vi "IG Create Error.vi"(4 "Skip Call Stack (1)":i32=1, 5 "Is Warning? (F)":bool, 6 "Name (Immediate Caller)":string, 7 "Show Call Chain? (T)":bool=TRUE, 8 "error in (no error)":errorcluster, 10 "Message (\"\")":string, 11 "Code":i32=1) -> (0 "error out":errorcluster)   [LabVIEW 2020, in "WS Admin.lvlib"]
uses:
  WS Admin.lvlib
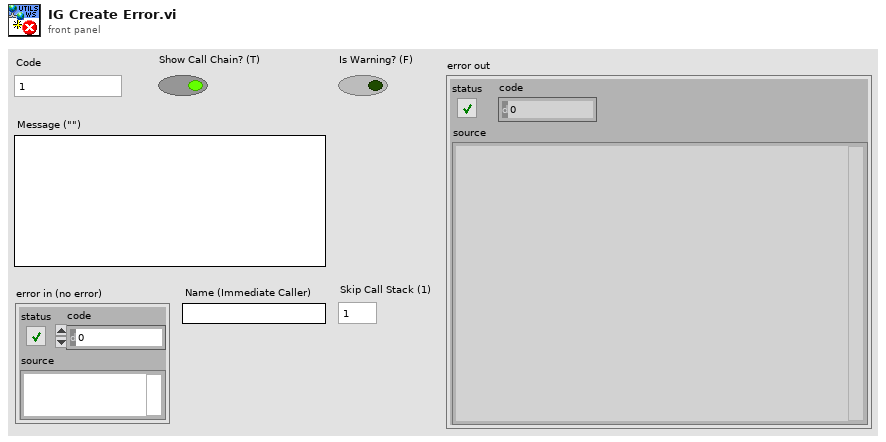
[diagram p1: front panel]
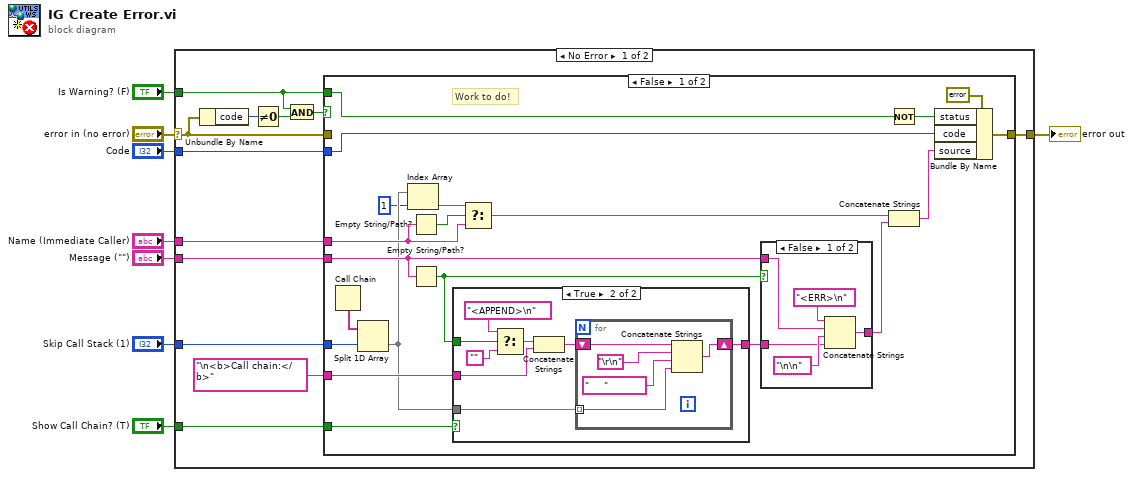
[diagram p0: block diagram]
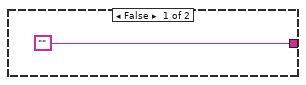
[diagram p3: hidden frame]
diagram:
  n1 = case shown="No Error" "error in (no error)" {
    selector: "error in (no error)" -> [w15 w62]
    tunnel: "Name (Immediate Caller)" -> [w20 _]
    tunnel: "Skip Call Stack (1)" -> [w19 _]
    tunnel: [w14 w62] -> w5
    tunnel: "Is Warning? (F)" -> [w13 _]
    tunnel: "Code" -> [w12 _]
    tunnel: "Show Call Chain? (T)" -> [w11 _]
    tunnel: "Message (\"\")" -> [w10 _]
    frame No Error {
      n2 = Unbundle By Name(w15) -> ("code"=w18:i32)
      n3 = Not Equal To 0?(x=w18) -> (x != 0?=w17:bool)
      n4 = And(x=w13, y=w17) -> (x .and. y?=w16:bool)
      n5 = case shown="False" w16 {
        tunnel: w20 -> [w38 _]
        tunnel: w19 -> [w23 _]
        tunnel: w15 -> [_ w61]
        tunnel: [w34 w61] -> w14
        tunnel: w13 -> [w32 _]
        tunnel: w12 -> [w33 _]
        tunnel: w11 -> [w31 _]
        tunnel: "\n<b>Call chain:</b>" ("call chain header") -> [w30 _]
        tunnel: w10 -> [w27 _]
        frame False {
          # "Work to do!"
          n6 = Call Chain() -> (call chain=w26:string[])
          n7 = Split 1D Array(array=w26, index=w23) -> (second subarray=w22:string[])  [unwired: 1 out]
          n8 = Index Array(array=w22, index=1) -> (element=w40:string)
          n9 = Empty String/Path?(string/path=w38) -> (empty?=w39:bool)
          n10 = Empty String/Path?(string/path=w27) -> (empty?=w28:bool)
          n11 = case shown="True" w31 {
            tunnel: w30 -> [_ w51]
            tunnel: w28 -> [_ w55]
            tunnel: ["" w50] -> w25
            tunnel: w22 -> [_ w48]
            frame False {
            }
            frame True {
              n12 = Select(t="<APPEND>\n", s=w55, f="") -> (s? t:f=w53:string)
              n13 = Concatenate Strings(w53, w51) -> (w52:string)
              n14 = for {
                shift-right: [w57] -> w50
                shift-left: w52 -> [w60]
                tunnel: w48 -> [w56] mode=indexing
                n15 = Concatenate Strings(w60, "\r\n", "     ", w56) -> (w57:string)
              }
            }
          }
          n16 = Select(t=w40, s=w39, f=w38) -> (s? t:f=w37:string)
          n17 = case shown="False" w28 {
            tunnel: w27 -> [w43 _]
            tunnel: w25 -> [w41 w46]
            tunnel: [w45 w46] -> w24
            frame False {
              n18 = Concatenate Strings("<ERR>\n", w43, "\n\n", w41) -> (w45:string)
            }
            frame True {
            }
          }
          n19 = Not(x=w32) -> (.not. x?=w35:bool)
          n20 = Concatenate Strings(w37, w24) -> (w29:string)
          n21 = Bundle By Name(cluster=errorcluster {"status"=FALSE, "code"=0, "source"=""} ("error constant"), "status"=w35, "code"=w33, "source"=w29) -> (w34:errorcluster)
        }
        frame True {
          # "Keep existing warning"
        }
      }
    }
    frame Error {
      # "Already an error, keep existing error."
    }
  }
  "error out" <- w5
